vi "Simulation Share.vi"() -> ()   [LabVIEW 2019, in "Thermostat Treiber.lvlib"]
uses:
  Thermostat Treiber.lvlib
panel:
  in  "Last Value":dbl
  in  "Abtastung":timestamp
  in  "Überlauf":timestamp
  in  "Temperatur":dbl
  in  "Rate":dbl
  in  "Last Update":timestamp
  in  "Ventil":dbl
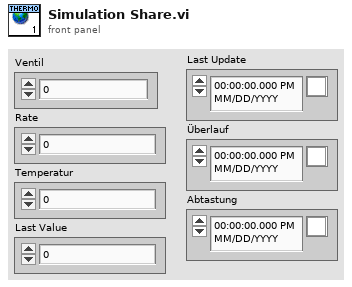
[diagram p1: front panel]
diagram:
